vi "test-translation2d.vi"(8 "error in (no error)":errorcluster) -> (0 "error out":errorcluster, 3 "All PASSED":bool)   [LabVIEW 2019]
uses:
  <vilib>/Rock Robotics/WPI/ThirdParty/JAS_Junk/TrajLib/TRANSLATION2D.ctl
  <vilib>/Rock Robotics/WPI/ThirdParty/JAS_Junk/TrajLib/Rotation_GetAngleCosSin.vi
  <vilib>/Rock Robotics/WPI/ThirdParty/JAS_Junk/TrajLib/Util_CalcDist.vi
  <vilib>/Rock Robotics/WPI/ThirdParty/JAS_Junk/TrajLib/Trajectory_Library.lvlib
panel:
  out "T10 X-7.79, Y=4.5":T1 {"Y" format="%14.3f"; "X" format="%14.3f"}
  out "T7 -- y -- 0":dbl
  out "T7 -- X -- 0":dbl
  out "T6 -- dist - 0":dbl
  out "T5 -- norm - 0":dbl
  out "T4 -- y -- 0":dbl
  out "T4 -- X -- 0":dbl
  out "T3 -- y -- 0":dbl
  out "T3 -- X -- 0":dbl
  out "T2 -- y -- 0":dbl
  out "T2 -- X -- 0":dbl
  out "T9 - False":bool
  out "T8 - True":bool
  out "T1 -- y -- 0":dbl
  out "T1 -- X -- 0":dbl
  out "T0 -- y -- 0":dbl
  out "T0 -- X -- 0":dbl
  # "Translation2D Test"
  # "Didn't implement divide"
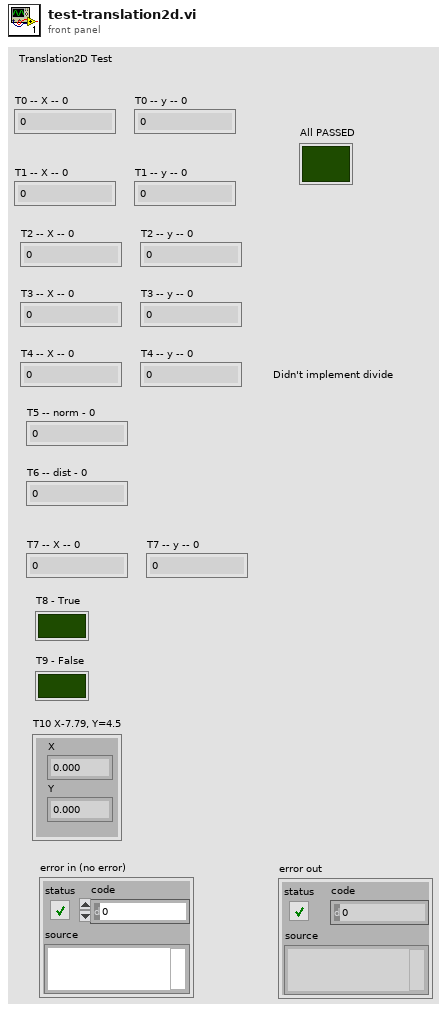
[diagram p1: front panel]
types:
  T1 = typedef "Trajectory_Library.lvlib/TRANSLATION2D.ctl" = cluster{"X":dbl, "Y":dbl}
  T2 = typedef "Trajectory_Library.lvlib/ROTATION2D.ctl" = cluster{"VALUE":dbl, "COS":dbl, "SIN":dbl}
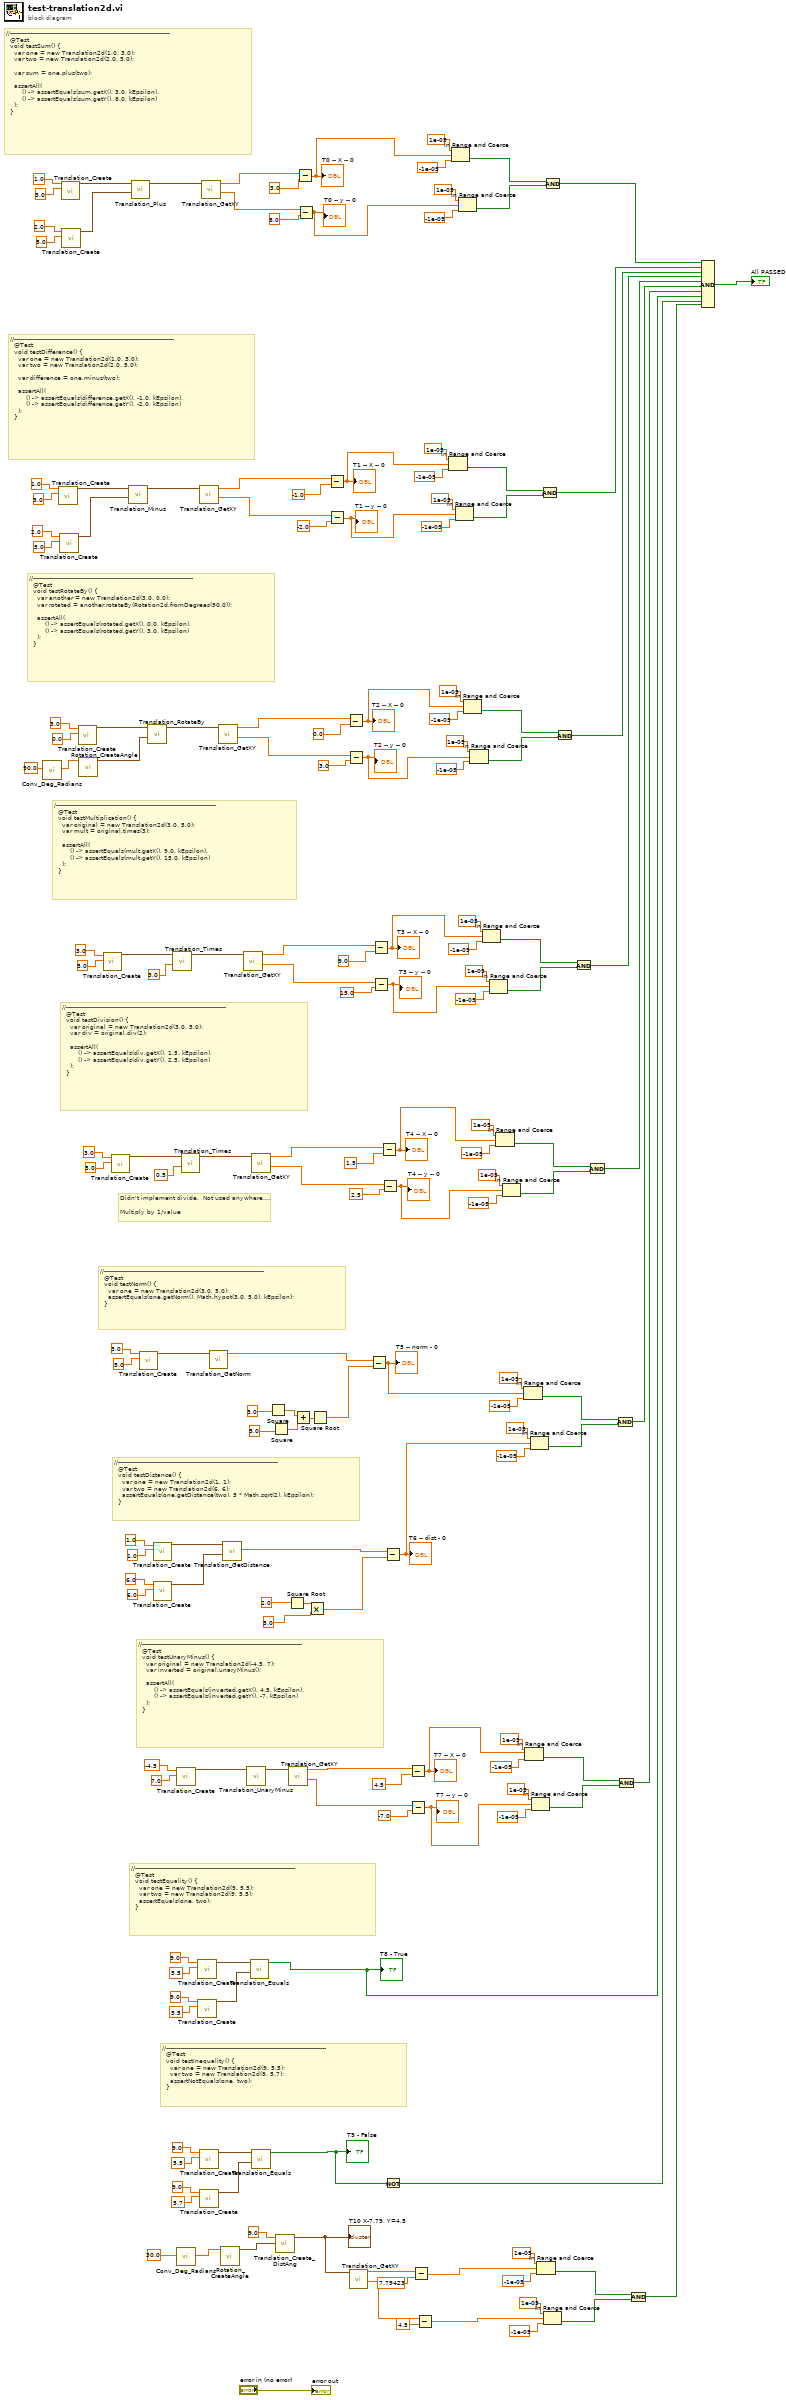
[diagram p0: block diagram]
diagram:
  # "//--------------------------------------------------------------------------------\n  @Test\n  void testInequality() {\n    var one = new Translation2d(9, 5.5);\n    var two = new Translation2d(9, 5.7);\n    assertNotEquals(one, two);\n  }"
  # "//--------------------------------------------------------------------------------\n  @Test\n  void testUnaryMinus() {\n    var original = new Translation2d(-4.5, 7);\n    var inverted = original.unaryMinus();\n\n    assertAll(\n        () -> assertEquals(inverted.getX(), 4.5, kEpsilon),\n        () -> assertEquals(inverted.getY(), -7, kEpsilon)\n    );\n  }"
  # "//--------------------------------------------------------------------------------\n  @Test\n  void testDistance() {\n    var one = new Translation2d(1, 1);\n    var two = new Translation2d(6, 6);\n    assertEquals(one.getDistance(two), 5 * Math.sqrt(2), kEpsilon);\n  }"
  # "//--------------------------------------------------------------------------------\n  @Test\n  void testNorm() {\n    var one = new Translation2d(3.0, 5.0);\n    assertEquals(one.getNorm(), Math.hypot(3.0, 5.0), kEpsilon);\n  }"
  # "Didn't implement divide.  Not used anywhere....\n\nMultiply by 1/value"
  # "//--------------------------------------------------------------------------------\n  @Test\n  void testDivision() {\n    var original = new Translation2d(3.0, 5.0);\n    var div = original.div(2);\n\n    assertAll(\n        () -> assertEquals(div.getX(), 1.5, kEpsilon),\n        () -> assertEquals(div.getY(), 2.5, kEpsilon)\n    );\n  }"
  # "/--------------------------------------------------------------------------------\n  @Test\n  void testMultiplication() {\n    var original = new Translation2d(3.0, 5.0);\n    var mult = original.times(3);\n\n    assertAll(\n        () -> assertEquals(mult.getX(), 9.0, kEpsilon),\n        () -> assertEquals(mult.getY(), 15.0, kEpsilon)\n    );\n  }"
  # "//--------------------------------------------------------------------------------\n  @Test\n  void testRotateBy() {\n    var another = new Translation2d(3.0, 0.0);\n    var rotated = another.rotateBy(Rotation2d.fromDegrees(90.0));\n\n    assertAll(\n        () -> assertEquals(rotated.getX(), 0.0, kEpsilon),\n        () -> assertEquals(rotated.getY(), 3.0, kEpsilon)\n    );\n  }"
  # "//--------------------------------------------------------------------------------\n  @Test\n  void testEquality() {\n    var one = new Translation2d(9, 5.5);\n    var two = new Translation2d(9, 5.5);\n    assertEquals(one, two);\n  }"
  # "//--------------------------------------------------------------------------------\n  @Test\n  void testDifference() {\n    var one = new Translation2d(1.0, 3.0);\n    var two = new Translation2d(2.0, 5.0);\n\n    var difference = one.minus(two);\n\n    assertAll(\n        () -> assertEquals(difference.getX(), -1.0, kEpsilon),\n        () -> assertEquals(difference.getY(), -2.0, kEpsilon)\n    );\n  }"
  # "//--------------------------------------------------------------------------------\n  @Test\n  void testSum() {\n    var one = new Translation2d(1.0, 3.0);\n    var two = new Translation2d(2.0, 5.0);\n\n    var sum = one.plus(two);\n\n    assertAll(\n        () -> assertEquals(sum.getX(), 3.0, kEpsilon),\n        () -> assertEquals(sum.getY(), 8.0, kEpsilon)\n    );\n  }"
  n1 = call <vilib>:"Conv_Deg_Radians.vi"("Degress"=90.0) -> ("Radians"=w148:dbl)  [unwired: 10 in]
  n2 = call <vilib>:"Translation_Create.vi"("Y"=3.0, "X"=1.0) -> ("TRANSLATION"=w162:T1)  [unwired: 9 in]
  n3 = call <vilib>:"Translation_Create.vi"("Y"=5.0, "X"=2.0) -> ("TRANSLATION"=w161:T1)  [unwired: 9 in]
  n4 = call <vilib>:"Translation_Create.vi"("Y"=3.0, "X"=1.0) -> ("TRANSLATION"=w171:T1)  [unwired: 9 in]
  n5 = call <vilib>:"Translation_Create.vi"("Y"=5.0, "X"=2.0) -> ("TRANSLATION"=w170:T1)  [unwired: 9 in]
  n6 = call <vilib>:"Translation_Create.vi"("Y"=0.0, "X"=3.0) -> ("TRANSLATION"=w153:T1)  [unwired: 9 in]
  n7 = call <vilib>:"Rotation_CreateAngle.vi"("Angle"=w148) -> ("ROTATION"=w146:T2)  [unwired: 10 in]
  n8 = call <vilib>:"Translation_Create.vi"("Y"=5.0, "X"=3.0) -> ("TRANSLATION"=w142:T1)  [unwired: 9 in]
  n9 = call <vilib>:"Translation_Create.vi"("Y"=5.0, "X"=3.0) -> ("TRANSLATION"=w133:T1)  [unwired: 9 in]
  n10 = call <vilib>:"Translation_Minus.vi"("other Translation"=w161, "In Translation"=w162) -> ("Out Translation"=w160:T1)  [unwired: 9 in]
  n11 = call <vilib>:"Translation_Plus.vi"("other Translation"=w170, "In Translation"=w171) -> ("Out Translation"=w169:T1)  [unwired: 9 in]
  n12 = call <vilib>:"Translation_Create.vi"("Y"=5.0, "X"=3.0) -> ("TRANSLATION"=w125:T1)  [unwired: 9 in]
  n13 = call <vilib>:"Translation_RotateBy.vi"("other Rotation"=w146, "In Translation"=w153) -> ("Out Translation"=w152:T1)  [unwired: 9 in]
  n14 = call <vilib>:"Translation_Create.vi"("Y"=1.0, "X"=1.0) -> ("TRANSLATION"=w115:T1)  [unwired: 9 in]
  n15 = call <vilib>:"Translation_Create.vi"("Y"=6.0, "X"=6.0) -> ("TRANSLATION"=w111:T1)  [unwired: 9 in]
  n16 = call <vilib>:"Translation_Times.vi"("Scalar"=3.0, "In Translation"=w142) -> ("Out Translation"=w141:T1)  [unwired: 9 in]
  n17 = call <vilib>:"Translation_Create.vi"("Y"=7.0, "X"=-4.5) -> ("TRANSLATION"=w104:T1)  [unwired: 9 in]
  n18 = call <vilib>:"Conv_Deg_Radians.vi"("Degress"=30.0 ("Y")) -> ("Radians"=w84:dbl)  [unwired: 10 in]
  n19 = call <vilib>:"Translation_Times.vi"("Scalar"=0.5, "In Translation"=w133) -> ("Out Translation"=w132:T1)  [unwired: 9 in]
  n20 = call <vilib>:"Translation_Create.vi"("Y"=5.5, "X"=9.0) -> ("TRANSLATION"=w94:T1)  [unwired: 9 in]
  n21 = call <vilib>:"Translation_Create.vi"("Y"=5.5, "X"=9.0) -> ("TRANSLATION"=w93:T1)  [unwired: 9 in]
  n22 = call <vilib>:"Translation_GetXY.vi"("In Translation"=w160) -> ("Y"=w158:dbl, "X"=w159:dbl)  [unwired: 9 in]
  n23 = call <vilib>:"Translation_Create.vi"("Y"=5.5, "X"=9.0) -> ("TRANSLATION"=w88:T1)  [unwired: 9 in]
  n24 = call <vilib>:"Translation_Create.vi"("Y"=5.7, "X"=9.0) -> ("TRANSLATION"=w87:T1)  [unwired: 9 in]
  n25 = call <vilib>:"Translation_GetXY.vi"("In Translation"=w169) -> ("Y"=w173:dbl, "X"=w174:dbl)  [unwired: 9 in]
  n26 = call <vilib>:"Translation_GetNorm.vi"("In Translation"=w125) -> ("Norm"=w119:dbl)  [unwired: 10 in]
  n27 = call <vilib>:"Translation_GetXY.vi"("In Translation"=w152) -> ("Y"=w150:dbl, "X"=w151:dbl)  [unwired: 9 in]
  n28 = call <vilib>:"Rotation_CreateAngle.vi"("Angle"=w84) -> ("ROTATION"=w85:T2)  [unwired: 10 in]
  n29 = call <vilib>:"Translation_GetDistance.vi"("other Translation"=w111, "In Translation"=w115) -> ("Distance"=w114:dbl)  [unwired: 9 in]
  n30 = call <vilib>:"Translation_GetXY.vi"("In Translation"=w141) -> ("Y"=w139:dbl, "X"=w140:dbl)  [unwired: 9 in]
  n31 = call <vilib>:"Translation_UnaryMinus.vi"("In Translation"=w104) -> ("Out Translation"=w101:T1)  [unwired: 10 in]
  n32 = call <vilib>:"Translation_Equals.vi"("other Translation"=w93, "In Translation"=w94) -> ("Equals"=w18:bool)  [unwired: 9 in]
  "T8 - True" <- w18
  n33 = call <vilib>:"Translation_GetXY.vi"("In Translation"=w132) -> ("Y"=w130:dbl, "X"=w131:dbl)  [unwired: 9 in]
  n34 = call <vilib>:"Translation_Equals.vi"("other Translation"=w87, "In Translation"=w88) -> ("Equals"=w17:bool)  [unwired: 9 in]
  "T9 - False" <- w17
  n35 = Square(x=3.0 ("X")) -> (x^2=w121:dbl)
  n36 = Square(x=5.0 ("X")) -> (x^2=w120:dbl)
  n37 = call <vilib>:"Translation_Create_DistAng.vi"("Angle"=w85, "Dist"=9.0 ("X")) -> ("TRANSLATION"=w9:T1)  [unwired: 9 in]
  "T10 X-7.79, Y=4.5" <- w9
  n38 = Square Root(x=2.0 ("X")) -> (sqrt(x)=w109:dbl)
  n39 = call <vilib>:"Translation_GetXY.vi"("In Translation"=w101) -> ("Y"=w99:dbl, "X"=w100:dbl)  [unwired: 9 in]
  n40 = Add(x=w121, y=w120) -> (x+y=w122:dbl)
  n41 = Subtract(x=w174, y=3.0) -> (x-y=w74:dbl)
  "T0 -- X -- 0" <- w74
  n42 = Subtract(x=w173, y=8.0) -> (x-y=w73:dbl)
  "T0 -- y -- 0" <- w73
  n43 = Multiply(x=w109, y=5.0 ("X")) -> (x*y=w107:dbl)
  n44 = Square Root(x=w122) -> (sqrt(x)=w118:dbl)
  n45 = Subtract(x=w159, y=-1.0 ("x")) -> (x-y=w66:dbl)
  "T1 -- X -- 0" <- w66
  n46 = Subtract(x=w158, y=-2.0) -> (x-y=w65:dbl)
  "T1 -- y -- 0" <- w65
  n47 = Subtract(x=w151, y=0.0 ("x")) -> (x-y=w57:dbl)
  "T2 -- X -- 0" <- w57
  n48 = Subtract(x=w150, y=3.0) -> (x-y=w56:dbl)
  "T2 -- y -- 0" <- w56
  n49 = call <vilib>:"Translation_GetXY.vi"("In Translation"=w9) -> ("Y"=w7:dbl, "X"=w8:dbl)  [unwired: 9 in]
  n50 = Subtract(x=w119, y=w118) -> (x-y=w30:dbl)
  "T5 -- norm - 0" <- w30
  n51 = Subtract(x=w140, y=9.0 ("x")) -> (x-y=w41:dbl)
  "T3 -- X -- 0" <- w41
  n52 = Subtract(x=w139, y=15.0) -> (x-y=w40:dbl)
  "T3 -- y -- 0" <- w40
  n53 = Subtract(x=w131, y=1.5 ("x")) -> (x-y=w39:dbl)
  "T4 -- X -- 0" <- w39
  n54 = Subtract(x=w130, y=2.5) -> (x-y=w38:dbl)
  "T4 -- y -- 0" <- w38
  n55 = Subtract(x=w114, y=w107) -> (x-y=w29:dbl)
  "T6 -- dist - 0" <- w29
  n56 = Not(x=w17) -> (.not. x?=w16:bool)
  n57 = Subtract(x=w100, y=4.5 ("x")) -> (x-y=w21:dbl)
  "T7 -- X -- 0" <- w21
  n58 = Subtract(x=w99, y=-7.0) -> (x-y=w20:dbl)
  "T7 -- y -- 0" <- w20
  n59 = Subtract(x=w8, y=7.79423) -> (x-y=w4:dbl)
  n60 = Subtract(x=w7, y=4.5) -> (x-y=w3:dbl)
  n61 = In Range and Coerce(upper limit=1e-05, x=w66, lower limit=-1e-05) -> (In Range?=w68:bool)  [unwired: 1 out]
  n62 = In Range and Coerce(upper limit=1e-05, x=w74, lower limit=-1e-05) -> (In Range?=w78:bool)  [unwired: 1 out]
  n63 = In Range and Coerce(upper limit=1e-05, x=w65, lower limit=-1e-05) -> (In Range?=w67:bool)  [unwired: 1 out]
  n64 = In Range and Coerce(upper limit=1e-05, x=w73, lower limit=-1e-05) -> (In Range?=w77:bool)  [unwired: 1 out]
  n65 = In Range and Coerce(upper limit=1e-05, x=w57, lower limit=-1e-05) -> (In Range?=w59:bool)  [unwired: 1 out]
  n66 = In Range and Coerce(upper limit=1e-05, x=w56, lower limit=-1e-05) -> (In Range?=w58:bool)  [unwired: 1 out]
  n67 = In Range and Coerce(upper limit=1e-05, x=w41, lower limit=-1e-05) -> (In Range?=w50:bool)  [unwired: 1 out]
  n68 = In Range and Coerce(upper limit=1e-05, x=w40, lower limit=-1e-05) -> (In Range?=w49:bool)  [unwired: 1 out]
  n69 = In Range and Coerce(upper limit=1e-05, x=w39, lower limit=-1e-05) -> (In Range?=w44:bool)  [unwired: 1 out]
  n70 = In Range and Coerce(upper limit=1e-05, x=w38, lower limit=-1e-05) -> (In Range?=w43:bool)  [unwired: 1 out]
  n71 = In Range and Coerce(upper limit=1e-05, x=w30, lower limit=-1e-05) -> (In Range?=w32:bool)  [unwired: 1 out]
  n72 = In Range and Coerce(upper limit=1e-05, x=w21, lower limit=-1e-05) -> (In Range?=w23:bool)  [unwired: 1 out]
  n73 = In Range and Coerce(upper limit=1e-05, x=w29, lower limit=-1e-05) -> (In Range?=w31:bool)  [unwired: 1 out]
  n74 = In Range and Coerce(upper limit=1e-05, x=w20, lower limit=-1e-05) -> (In Range?=w22:bool)  [unwired: 1 out]
  n75 = In Range and Coerce(upper limit=1e-05, x=w4, lower limit=-1e-05) -> (In Range?=w11:bool)  [unwired: 1 out]
  n76 = Compound Arithmetic op=AND(w68, w67) -> (w64:bool)
  n77 = In Range and Coerce(upper limit=1e-05, x=w3, lower limit=-1e-05) -> (In Range?=w10:bool)  [unwired: 1 out]
  n78 = Compound Arithmetic op=AND(w78, w77) -> (w76:bool)
  n79 = Compound Arithmetic op=AND(w59, w58) -> (w55:bool)
  n80 = Compound Arithmetic op=AND(w50, w49) -> (w42:bool)
  n81 = Compound Arithmetic op=AND(w44, w43) -> (w37:bool)
  n82 = Compound Arithmetic op=AND(w32, w31) -> (w28:bool)
  n83 = Compound Arithmetic op=AND(w23, w22) -> (w19:bool)
  n84 = Compound Arithmetic op=AND(w11, w10) -> (w2:bool)
  n85 = Compound Arithmetic op=AND(w76, w64, w55, w42, w37, w28, w19, w18, w16, w2) -> (→"All PASSED":bool)
  "error out" <- "error in (no error)"
